vi "Perform measurement.vi"(6 "measurement configuration":T4={"Victim channel"=0, "Full scale range"=10.0, "Interferer channels"=[2], "Victim channel resource name"="", "Victim frequency"=1000.0, "Victim amplitude"=-1.0, "Interferer channel resource name"="", "Interferer channel channel"=0, "Interferer start frequency"=100000.0, "Interferer stop frequency"=160000.0, "Interferer number of steps"=10, "Interferer sweep type"=0, "Interferer amplitude"=-1.0, "Digital capture resource name"="", "Digital capture sample rate"=800000.0, "Digital capture samples"=800000} {"Interferer sweep type" items=["Linear", "Logarithmic"]}, 7 "Measurement Context":refnum<class "Measure Call Context.lvclass">, 11 "device sessions":T2) -> (0 "error out":errorcluster, 2 "measurement results":T3)   [LabVIEW 2021, in "Channel To Channel Isolation_ADC.lvlib"]
uses:
  Channel To Channel Isolation_ADC.lvlib
  Measurement Configuration.ctl
  Measurement Results.ctl
  <vilib>/MeasurementLink/MeasurementLink Measurement Server/Measure Call Context/Measure Call Context.lvclass
  <vilib>/gRPC/LabVIEW gRPC Library/Shared/grpcId.ctl
  <vilib>/Analysis/1siggen.llb/Ramp Pattern by Samples.vi
  <vilib>/addons/_NISVFA/_Shared subVIs/Common/SVL Set dB Reference (N Ch - 1 Ref).vi
  <vilib>/addons/_NISVFA/_Shared subVIs/Common/SVL Set dB Reference (1 Ch).vi
  <vilib>/addons/_NISVFA/_Shared subVIs/Common/SVL Set dB Reference (variant).vi
  <vilib>/MeasurementLink/MeasurementLink Measurement Server/Measure Call Context/Accessor/Is Canceled.vi
  <vilib>/addons/_NISVFA/_Shared subVIs/Common/svc_Caller VI Returned in Error Source.vi
  <vilib>/Analysis/NI_AALBase.lvlib
  shared/digitalInterface/client/dcvmDPI_AD7606B_clientImpl/dcvmDPI_AD7606B_clientImpl.lvlib
  <vilib>/gRPC/LabVIEW gRPC Library/grpc-lvsupport-release.lvlib
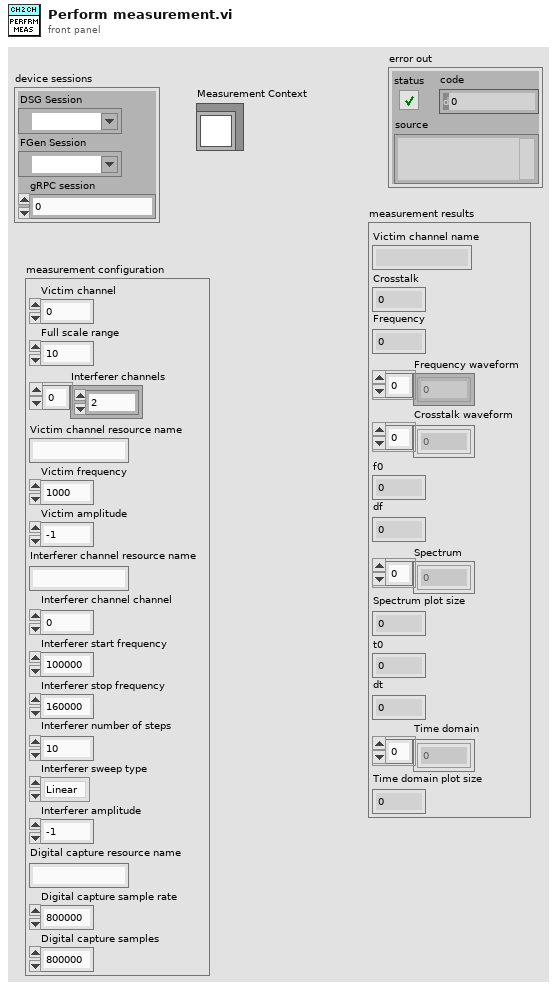
[diagram p1: front panel]
types:
  T1 = typedef "grpc-lvsupport-release.lvlib/grpcId.ctl" = u64
  T2 = cluster{"DSG Session":refnum<k21>, "FGen Session":refnum<k15>, "gRPC session":T1}
  T3 = typedef "Channel To Channel Isolation_ADC.lvlib/Measurement Results.ctl" = cluster{"Victim channel name":string, "Crosstalk":dbl, "Frequency":dbl, "Frequency waveform":dbl[], "Crosstalk waveform":dbl[], "f0":dbl, "df":dbl, "Spectrum":dbl[], "Spectrum plot size":i32, "t0":dbl, "dt":dbl, "Time domain":dbl[], "Time domain plot size":i32}
  T4 = typedef "Channel To Channel Isolation_ADC.lvlib/Measurement Configuration.ctl" = cluster{"Victim channel":i32, "Full scale range":dbl, "Interferer channels":i32[], "Victim channel resource name":string, "Victim frequency":dbl, "Victim amplitude":dbl, "Interferer channel resource name":string, "Interferer channel channel":i32, "Interferer start frequency":dbl, "Interferer stop frequency":dbl, "Interferer number of steps":i32, "Interferer sweep type":u32, "Interferer amplitude":dbl, "Digital capture resource name":string, "Digital capture sample rate":dbl, "Digital capture samples":u32}
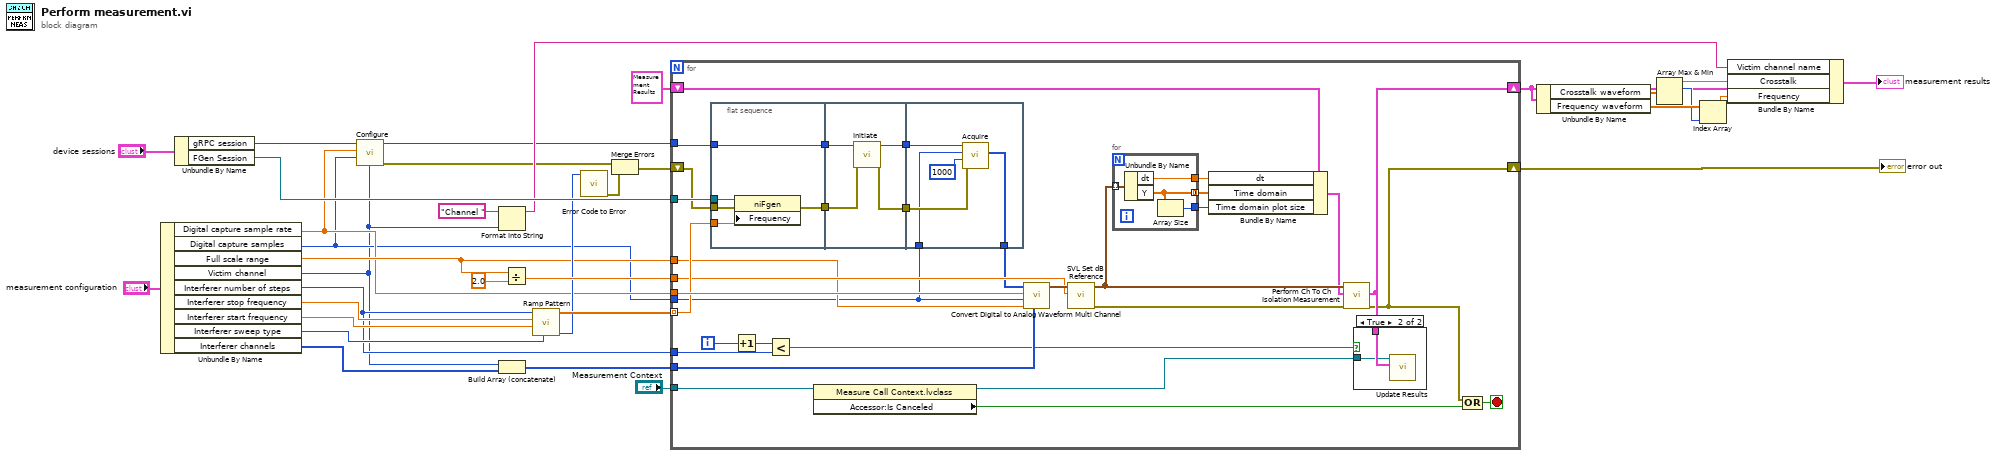
[diagram p0: block diagram]
diagram:
  n1 = Unbundle By Name("measurement configuration") -> ("Digital capture sample rate"=w5:dbl, "Digital capture samples"=w4:u32, "Full scale range"=w13:dbl, "Victim channel"=w3:i32, "Interferer number of steps"=w8:i32, "Interferer stop frequency"=w32:dbl, "Interferer start frequency"=w31:dbl, "Interferer sweep type"=w9:u32, "Interferer channels"=w26:i32[])
  n2 = Unbundle By Name("device sessions") -> ("gRPC session"=w6:T1, "FGen Session"=w29:refnum<k15>)
  n3 = call "Configure.vi"("Input channel"=w3, "Digital capture samples"=w4, "Digital capture sample rate"=w5, "gRPC session in"=w6) -> ("error out"=w1:errorcluster, "gRPC session out"=w2:T1)  [unwired: 6 in]
  n4 = Format Into String(initial string="Channel ", w3) -> (resulting string=w11:string)  [unwired: 2 in, 1 out]
  n5 = Build Array (concatenate)(w3, w26) -> (w25:i32[])
  n6 = Divide(x=w13, y=2.0) -> (x/y=w27:dbl)
  n7 = call-poly <vilib>:"Ramp Pattern.vi"("type"=w9, "start"=w31, "end"=w32, "samples"=w8) -> ("error"=w16:i32, "Ramp Pattern"=w30:dbl[])  [unwired: 6 in]
  n8 = call "Error Code to Error.vi"("error code"=w16) -> ("error"=w15:errorcluster)  [unwired: 10 in]
  n9 = Merge Errors(w1, w15) -> (w14:errorcluster)
  n10 = for {
    tunnel: w4 -> [w36]
    tunnel: w5 -> [w66]
    shift-right: [w45] -> w24
    shift-left: w14 -> [w63]
    tunnel: w30 -> [w64] mode=indexing
    tunnel: w29 -> [w65]
    tunnel: w27 -> [w61]
    tunnel: w25 -> [w60]
    shift-right: [w51] -> w19
    shift-left: T3 {"Victim channel name"="", "Crosstalk"=0.0, "Frequency"=0.0, "Frequency waveform"=[], "Crosstalk waveform"=[], "f0"=0.0, "df"=0.0, "Spectrum"=[], "Spectrum plot size"=0, "t0"=0.0, "dt"=0.0, "Time domain"=[], "Time domain plot size"=0} ("Measurement Results out") -> [w55]
    tunnel: w13 -> [w52]
    tunnel: "Measurement Context" -> [w46]
    tunnel: w8 -> [w42]
    tunnel: w2 -> [w40]
    i -> [w50]
    stop <- w43 stop-if-true
    n11 = flat-sequence {
      tunnel: w65 -> [w71]
      tunnel: w64 -> [w70]
      tunnel: w63 -> [w69]
      tunnel: [w68] -> w41
      tunnel: w40 -> [w68]
      tunnel: [w67] -> w39
      tunnel: w41 -> [w75]
      tunnel: w39 -> [w74]
      tunnel: [w73] -> w38
      tunnel: [w72] -> w37
      tunnel: w38 -> [w79]
      tunnel: w37 -> [w80]
      tunnel: w36 -> [w78]
      tunnel: [w76] -> w35
      frame #0 {
        n12 = property class="niFgen"(reference=w71, error in=w69, "Frequency"=w70) -> (error out=w67:errorcluster)  [unwired: 1 out]
      }
      frame #1 {
        n13 = call "Initiate.vi"("error in"=w74, "gRPC session in"=w75) -> ("error out"=w73:errorcluster, "gRPC session out"=w72:T1)  [unwired: 8 in]
      }
      frame #2 {
        n14 = call "Acquire.vi"("error in"=w79, "Timeout (ms)"=1000, "Digital capture samples"=w78, "gRPC session in"=w80) -> ("Digital waveform"=w76:u32[])  [unwired: 5 in, 2 out]
      }
    }
    n15 = Increment(x=w50) -> (x+1=w49:i32)
    n16 = Less?(x=w49, y=w42) -> (x < y?=w48:bool)
    n17 = property class="Measure Call Context.lvclass"(reference=w46) -> (reference out=w47:refnum<class "Measure Call Context.lvclass">, "Accessor:Is Canceled"=w44:bool)  [unwired: 1 in, 1 out]
    n18 = call "Convert Digital to Analog Waveform Multi Channel.vi"("Channels index"=w60, "full scale range"=w52, "Number of samples"=w36, "Sample rate"=w66, "Digital Waveform"=w35) -> ("Waveforms"=w62:waveform(dbl)[])  [unwired: 6 in]
    n19 = call-poly <vilib>:"SVL Set dB Reference.vi"("dB reference [EU]"=w61, "scaled signals in [EU]"=w62) -> ("error out"=w59:errorcluster, "scaled signals out [EU]"=w58:waveform(dbl)[])  [unwired: 8 in]
    n20 = for {
      tunnel: w58 -> [w86] mode=indexing
      tunnel: [w84] -> w57 mode=concatenating
      tunnel: [w85] -> w56
      tunnel: [w83] -> w53
      n21 = Unbundle By Name(w86) -> ("dt"=w85:dbl, "Y"=w84:dbl[])
      n22 = Array Size(array=w84) -> (size(s)=w83:i32)
    }
    n23 = Bundle By Name(cluster=w55, "dt"=w56, "Time domain"=w57, "Time domain plot size"=w53) -> (w54:T3)
    n24 = call "Perform Ch To Ch Isolation Measurement.vi"("error in"=w59, "Measurement Results in"=w54, "ananlog waveforms"=w58) -> ("error out"=w45:errorcluster, "Measurement Results out"=w51:T3)  [unwired: 7 in]
    n25 = case shown="True" w48 {
      tunnel: w51 -> [_ w82]
      tunnel: w47 -> [_ w81]
      frame False {
      }
      frame True {
        n26 = call <vilib>:"Update Results.vi"("measurement results"=w82, "measure call context in"=w81) -> ()  [unwired: 8 in, 2 out]
      }
    }
    n27 = Compound Arithmetic op=OR(w45, w44) -> (w43:bool)
  }
  "error out" <- w24
  n28 = Unbundle By Name(w19) -> ("Crosstalk waveform"=w23:dbl[], "Frequency waveform"=w22:dbl[])
  n29 = Array Max & Min(array=w23) -> (max value=w17:dbl, max index (indices)=w21:i32)  [unwired: 2 out]
  n30 = Index Array(array=w22, index=w21) -> (element=w20:dbl)
  n31 = Bundle By Name(cluster=w19, "Victim channel name"=w11, "Crosstalk"=w17, "Frequency"=w20) -> (→"measurement results":T3)
